vi "GetGrowableReference.vi"(8 "error in":errorcluster, 11 "Function in":refnum<class "GrowableFunction.lvclass">) -> (0 "error out":errorcluster, 1 "reference out":refnum<vi>, 3 "Function out":refnum<class "GrowableFunction.lvclass">)   [LabVIEW 2014, in "Raspberry Pi Compatible Compiler for LabVIEW.lvlib" / "GrowableFunction.lvclass"]
uses:
  GrowableFunction.lvclass
  Generic/Generic.lvclass
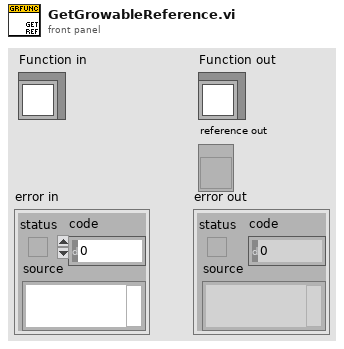
[diagram p1: front panel]
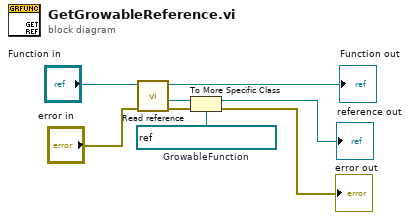
[diagram p0: block diagram]
diagram:
  w5 = refnum<vi> refnum  # GrowableFunction
  n1 = call "Read reference.vi"("error in"="error in", "GObject in"="Function in") -> ("error out"=w6:errorcluster, "reference"=w7:refnum<vi>, "GObject out"=→"Function out":refnum<class "GrowableFunction.lvclass">)  [unwired: 5 in]
  n2 = To More Specific Class(target class=w5, reference=w7, error in=w6) -> (specific class reference=→"reference out":refnum<vi>, error out=→"error out":errorcluster)
